vi "coils dataframe.vi"() -> ()   [LabVIEW 2015]
uses:
  <vilib>/Utility/config.llb/NI_LVConfig.lvlib
panel:
  out "数组－数值":u16[](array[numeric])
  out "起始地址 2":string caption="0x"
  in  "线圈数量":u32 max=2000 format="%04d"
  in  "起始地址":u16 format="%04x"
  in  "Coils":bool[][](array[boolean])
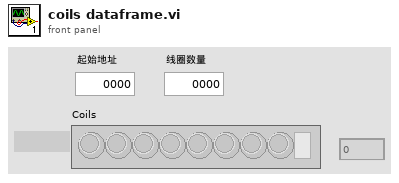
[diagram p1: front panel]
types:
  T1 = typedef "LVRectTypeDef.ctl" = cluster{"Left":i16, "Top":i16, "Right":i16, "Bottom":i16}
  T2 = typedef "LVPointTypeDef.ctl" = cluster{"Horizontal":i16, "Vertical":i16}
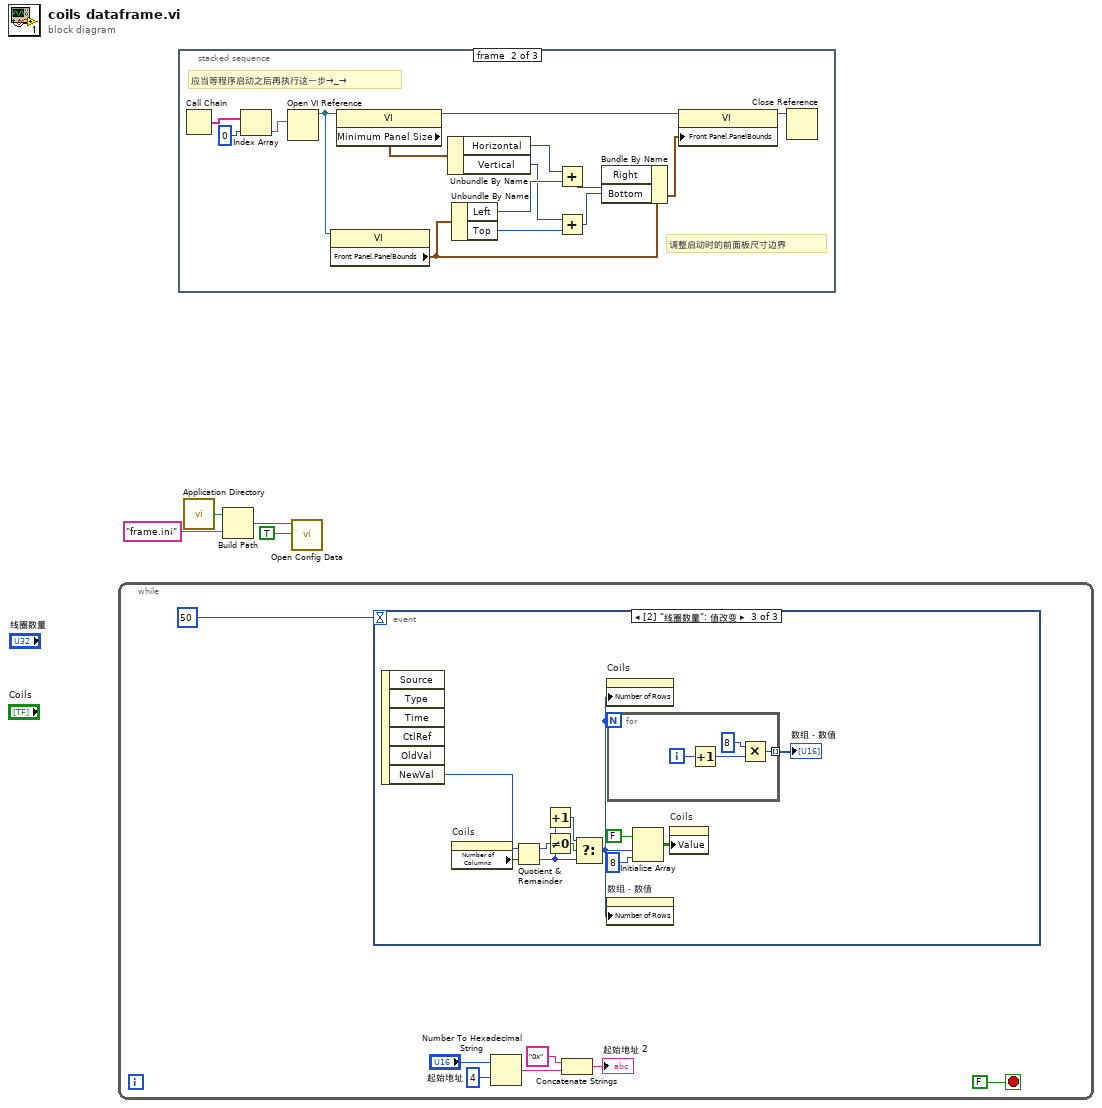
[diagram p0: block diagram]
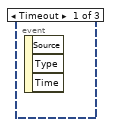
[diagram p2: hidden frame]
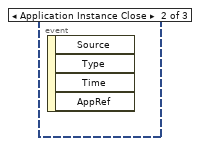
[diagram p3: hidden frame]
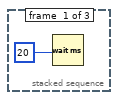
[diagram p4: hidden frame]
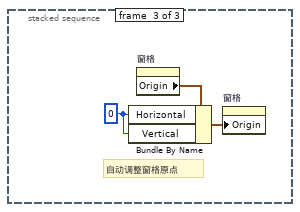
[diagram p5: hidden frame]
diagram:
  n1 = while {
    stop <- FALSE stop-if-true
    n2 = event shown="[2] \"线圈数量\": 值改变" {
      selector: _ -> [_ _ _]
      dyn-events: _ -> [_ _ _]
      timeout: 50 -> [_ _ _]
      event Timeout {
        n3 = event-data() -> ()  [unwired: 1 in, 3 out]
      }
      event Application Instance Close {
        n4 = event-data() -> ()  [unwired: 1 in, 4 out]
      }
      event "线圈数量": Value Change {
        n5 = event-data() -> ("NewVal"=w22:u32)  [unwired: 1 in, 5 out]
        n6 = property on="Coils" class="Arr (严格)"() -> ("Number of Columns"=w21:u32)  [unwired: 2 in, 2 out]
        n7 = Quotient & Remainder(x=w22, y=w21) -> (x-y*floor(x/y)=w20:u32, floor(x/y)=w17:u32)
        n8 = Increment(x=w17) -> (x+1=w18:u32)
        n9 = Not Equal To 0?(x=w20) -> (x != 0?=w19:bool)
        n10 = Select(t=w18, s=w19, f=w17) -> (s? t:f=w13:u32)
        n11 = property on="Coils" class="Arr (严格)"("Number of Rows"=w13) -> ()  [unwired: 2 in, 2 out]
        n12 = for {
          N: w13 -> [_]
          tunnel: [w25] -> w12 mode=indexing
          i -> [w26]
          n13 = Increment(x=w26) -> (x+1=w24:i32)
          n14 = Multiply(x=u16 8, y=w24) -> (x*y=w25:i32)
        }
        "数组－数值" <- w12
        n15 = property on="数组－数值" class="Arr (严格)"("Number of Rows"=w13) -> ()  [unwired: 2 in, 2 out]
        n16 = Initialize Array(FALSE, w13, 8) -> (w15:bool[][])
        n17 = property on="Coils" class="Arr (严格)"("Value"=w15) -> ()  [unwired: 2 in, 2 out]
      }
    }
    n18 = Number To Hexadecimal String(1:4, 2:"起始地址") -> (0:w7:string)
    n19 = Concatenate Strings("0x", w7) -> (→"起始地址 2":string)
  }
  n20 = stacked-sequence {
    frame #0 {
      n21 = Wait (ms)(milliseconds to wait=u32 20) -> ()  [unwired: 1 out]
    }
    frame #1 {
      # "调整启动时的前面板尺寸边界"
      # "应当等程序启动之后再执行这一步→_→"
      n22 = Call Chain ("调用链")() -> (call chain=w30:string[])
      n23 = Index Array(array=w30, index=0) -> (element=w28:string)
      n24 = Open VI Reference(vi path=w28) -> (vi reference=w40:refnum<vi>)  [unwired: 1 in, 5 out]
      n25 = property class="VI"(reference=w40) -> ("Front Panel.PanelBounds"=w37:T1)  [unwired: 1 in, 2 out]
      n26 = property class="VI"(reference=w40) -> (reference out=w41:refnum<vi>, "Minimum Panel Size"=w31:T2)  [unwired: 1 in, 1 out]
      n27 = Unbundle By Name(w31) -> ("Horizontal"=w38:i16, "Vertical"=w35:i16)
      n28 = Unbundle By Name(w37) -> ("Left"=w39:i16, "Top"=w34:i16)
      n29 = Add(x=w38, y=w39) -> (x+y=w36:i16)
      n30 = Add(x=w35, y=w34) -> (x+y=w33:i16)
      n31 = Bundle By Name(cluster=w37, "Right"=w36, "Bottom"=w33) -> (w32:T1)
      n32 = property class="VI"(reference=w41, "Front Panel.PanelBounds"=w32) -> (reference out=w42:refnum<vi>)  [unwired: 1 in, 1 out]
      n33 = Close Reference(reference=w42) -> ()  [unwired: 1 in, 1 out]
    }
    frame #2 {
      w45 = i16 0
      # "自动调整窗格原点"
      n34 = property on="窗格" class="Pane"() -> ("Origin"=w44:T2)  [unwired: 2 in, 2 out]
      n35 = Bundle By Name(cluster=w44, "Horizontal"=w45, "Vertical"=w45) -> (w43:T2)
      n36 = property on="窗格" class="Pane"("Origin"=w43) -> ()  [unwired: 2 in, 2 out]
    }
  }
  n37 = call <vilib>:"Application Directory.vi"() -> ("Application Directory"=w3:path)
  n38 = Build Path(base path=w3, name or relative path="frame.ini") -> (appended path=w2:path)
  n39 = call <vilib>:"Open Config Data.vi"("create file if necessary (T)"=TRUE, "configuration file path"=w2) -> ()  [unwired: 7 in, 3 out]
